vi "dashboard_globals.vi"() -> ()   [LabVIEW 2011]
panel:
  in  "battery":dbl
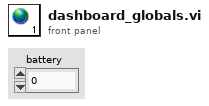
[diagram p1: front panel]
diagram:
